vi "RDS Serial Handler Send Frame.vi"(8 "error in (no error)":errorcluster, 10 "Serial Frame":refnum<class "RDS Serial Frame.lvclass">, 11 "RDS Serial Instrument in":refnum<class "RDS Serial Instrument.lvclass">) -> (0 "error out":errorcluster, 3 "RDS Serial Instrument out":refnum<class "RDS Serial Instrument.lvclass">)   [LabVIEW 2015, in "RDS Serial Handler.lvlib" / "RDS Serial Instrument.lvclass"]
uses:
  RDS Serial Instrument.lvclass
  RDS Serial Frame.lvclass
  RDS Serial Instrument.lvclass/RDS Serial Instrument.ctl
  RDS Serial Frame.lvclass/RDS Serial Frame.ctl
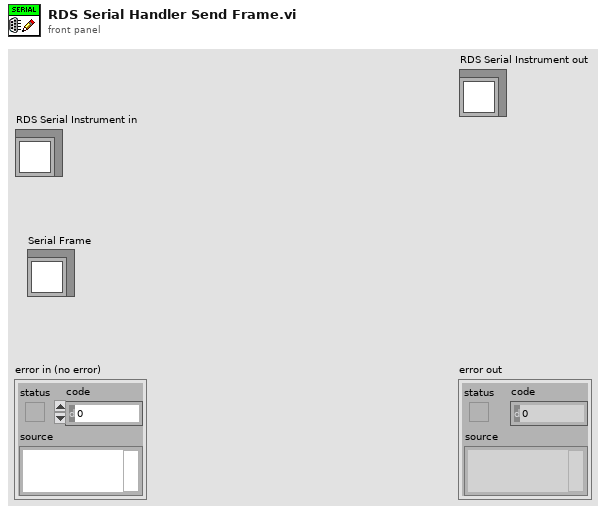
[diagram p1: front panel]
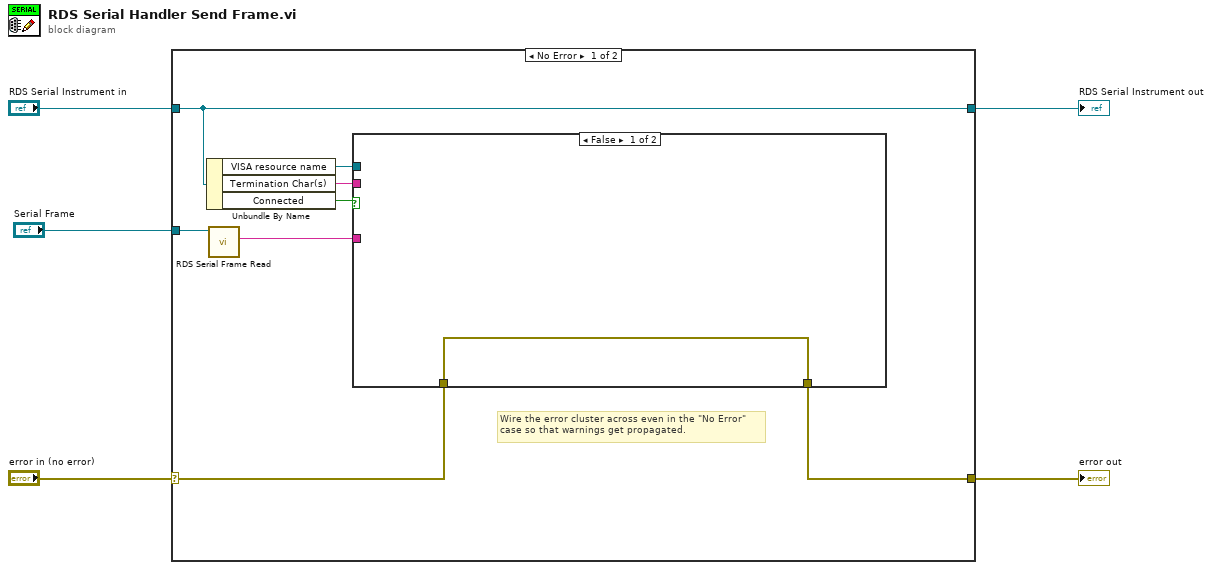
[diagram p0: block diagram]
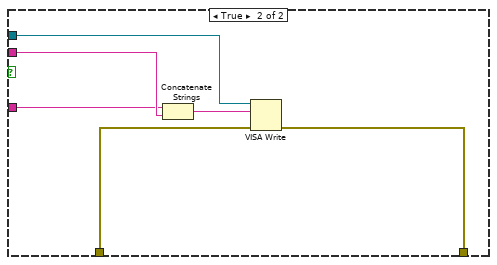
[diagram p2: hidden frame]
diagram:
  n1 = case shown="No Error" "error in (no error)" {
    selector: "error in (no error)" -> [w11 w22]
    tunnel: [w10 w22] -> w4
    tunnel: [w13 w21] -> w2
    tunnel: "RDS Serial Instrument in" -> [w13 w21]
    tunnel: "Serial Frame" -> [w8 _]
    frame No Error {
      # "Wire the error cluster across even in the \"No Error\"\ncase so that warnings get propagated."
      n2 = Unbundle By Name(w13) -> ("VISA resource name"=w12:refnum<visa-resource-name>, "Termination Char(s)"=w9:string, "Connected"=w6:bool)
      n3 = call "RDS Serial Frame Read.vi"("RDS Serial Frame in"=w8) -> ("Serial String"=w7:string)  [unwired: 7 in, 3 out]
      n4 = case shown="False" w6 {
        tunnel: w12 -> [_ w20]
        tunnel: w11 -> [w14 w19]
        tunnel: [w14 w18] -> w10
        tunnel: w9 -> [_ w17]
        tunnel: w7 -> [_ w15]
        frame False {
        }
        frame True {
          n5 = Concatenate Strings(w15, w17) -> (w16:string)
          n6 = VISA Write(VISA resource name=w20, write buffer=w16, error in (no error)=w19) -> (error out=w18:errorcluster)  [unwired: 2 out]
        }
      }
    }
    frame Error {
    }
  }
  "error out" <- w4
  "RDS Serial Instrument out" <- w2
